vi "SendAOProtocol.vi"(7 "Send":bool, 9 "Initialize":bool, 10 "prev":T1={"type"="AO", "device"="", "name"="", "data"={"<init"=FALSE, "<voltage"=0.0}}, 11 "new":T1={"type"="AO", "device"="", "name"="", "data"={"<init"=FALSE, "<voltage"=0.0}}) -> ()   [LabVIEW 2019]
uses:
  AO proto.ctl
  AO Data proto.ctl
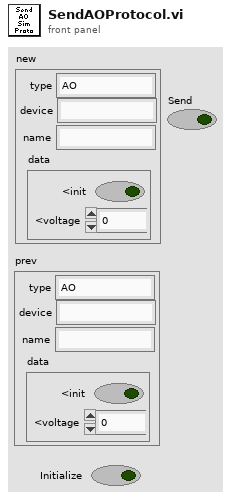
[diagram p1: front panel]
types:
  T1 = typedef "AO proto.ctl" = cluster{"type":string, "device":string, "name":string, "data":T2}
  T2 = typedef "AO Data proto.ctl" = cluster{"<init":bool, "<voltage":dbl}
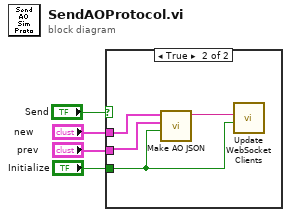
[diagram p0: block diagram]
diagram:
  n1 = case shown="True" "Send" {
    tunnel: "new" -> [_ w6]
    tunnel: "prev" -> [_ w7]
    tunnel: "Initialize" -> [_ w5]
    frame False {
    }
    frame True {
      n2 = call "Make AO JSON.vi"("Force"=w5, "AO prev"=w7, "AO new"=w6) -> ("delta JSON"=w8:string)  [unwired: 8 in]
      n3 = call "Update WebSocket Clients.vi"("Initialize"=w5, "delta JSON"=w8) -> ()  [unwired: 10 in]
    }
  }
